vi "se2.vi"() -> ()   [LabVIEW 2013]
panel:
  out "Numeric":i32
  in  "Knob":dbl(knob) scale=0.0..2.0
  out "Waveform Chart":dbl(graph)
  in  "Boolean":bool
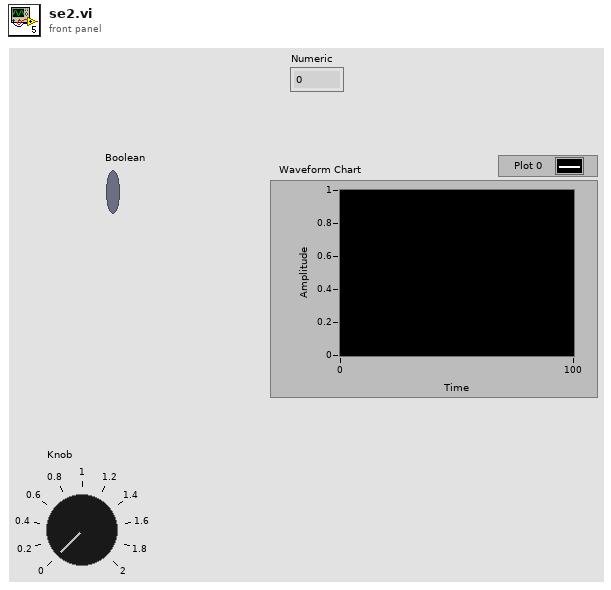
[diagram p1: front panel]
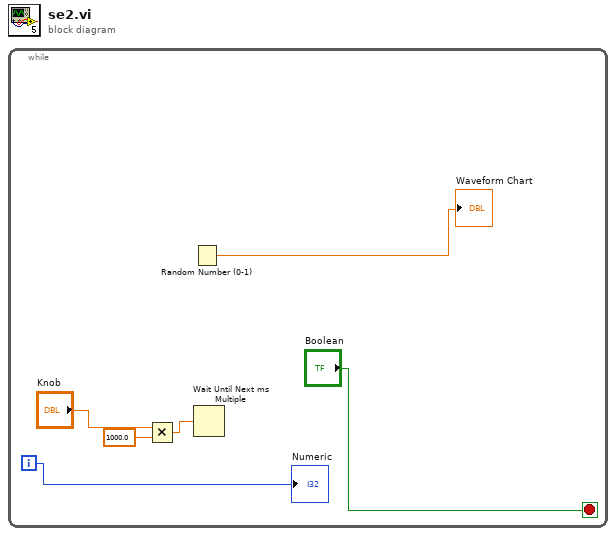
[diagram p0: block diagram]
diagram:
  n1 = while {
    i -> [w3]
    stop <- "Boolean" stop-if-true
    n2 = Multiply(x="Knob", y=1000.0) -> (x*y=w5:dbl)
    n3 = Random Number (0-1)() -> (number: 0 to 1=→"Waveform Chart":dbl)
    n4 = Wait Until Next ms Multiple(millisecond multiple=w5) -> ()  [unwired: 1 out]
    "Numeric" <- w3
  }
